vi "Read System Status.vi"(8 "Error in":errorcluster caption="错误输入", 10 "Channel":dbl=1.0 caption="设备通道", 11 "Modbus master in":refnum<class "Modbus Master.lvclass"> caption="Modbus实例输入") -> (0 "Error out":errorcluster caption="错误输出", 1 "Run Status Information":string caption="运行状态信息", 2 "Error Information":string caption="错误信息", 3 "Modbus instance out":refnum<class "Modbus API.lvclass"> caption="Modbus实例输出")   [LabVIEW 2023, in "Longer Pump dLSP501 Series.lvlib"]
uses:
  <instrlib>/Longer Pump dLSP501 Modbus RTU Series/Longer Pump dLSP501 Series.lvlib
  <vilib>/NI/Modbus Library/API/Modbus API.lvclass
  <vilib>/NI/Modbus Library/API/Master/Modbus Master.lvclass
  C:/Program Files/National Instruments/LabVIEW 2023/vi.lib/NI/Modbus Library/API/Modbus API.lvclass
panel:
  out "Register Values":u16[](array[numeric]) caption="寄存器值"
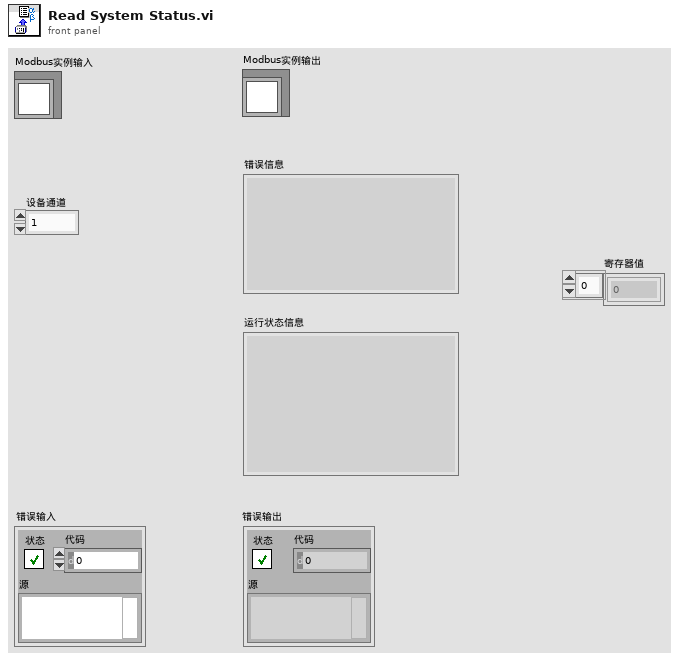
[diagram p1: front panel]
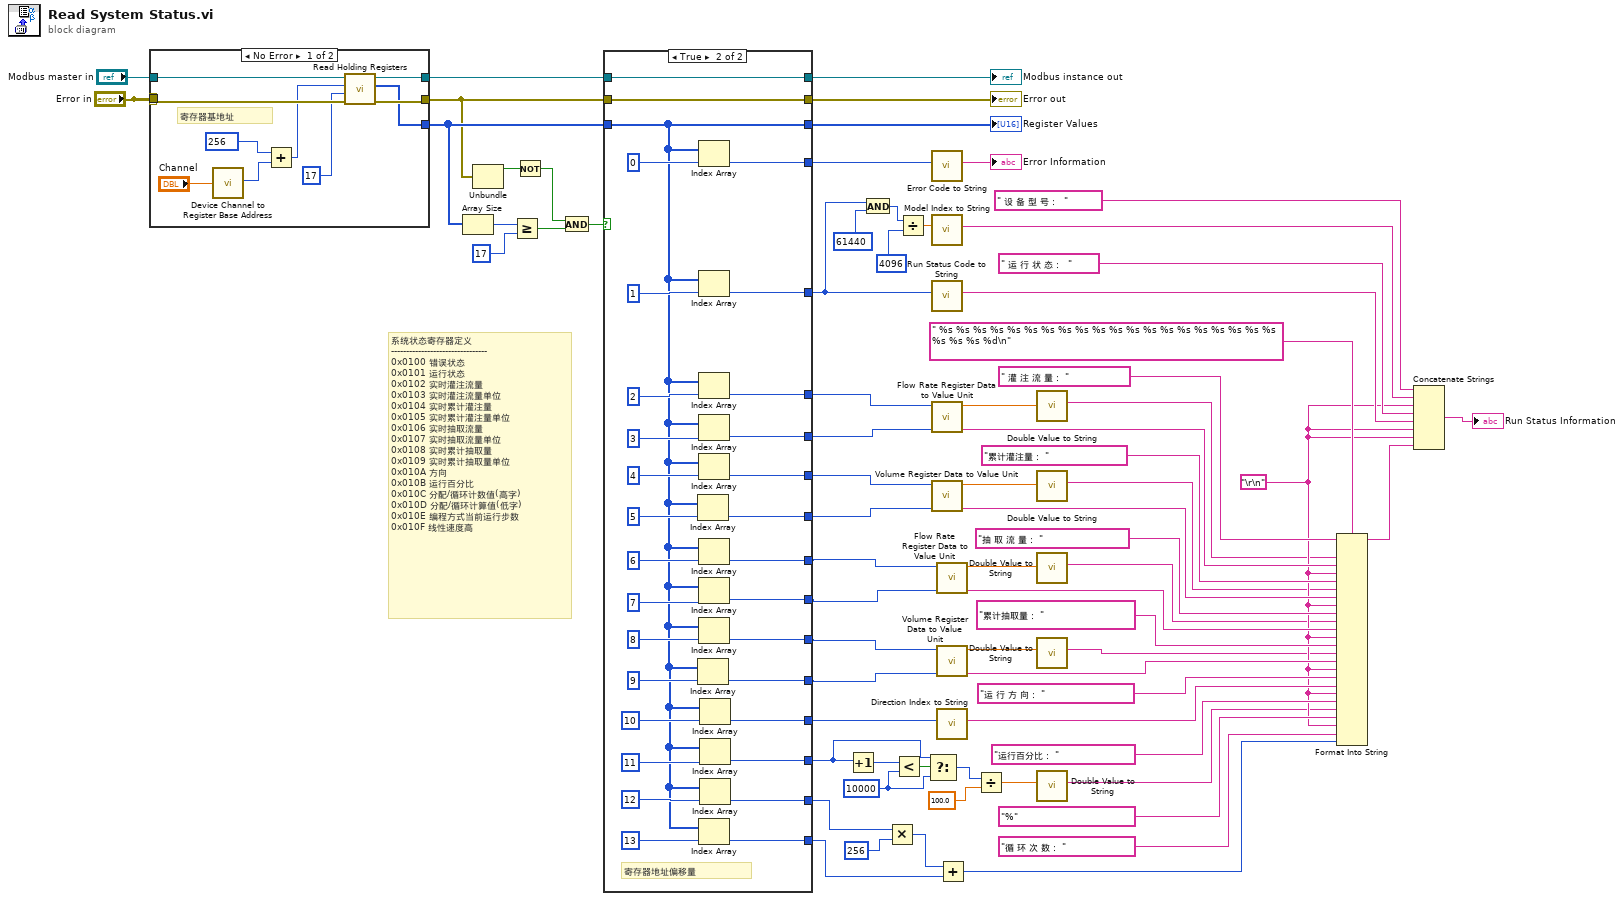
[diagram p0: block diagram]
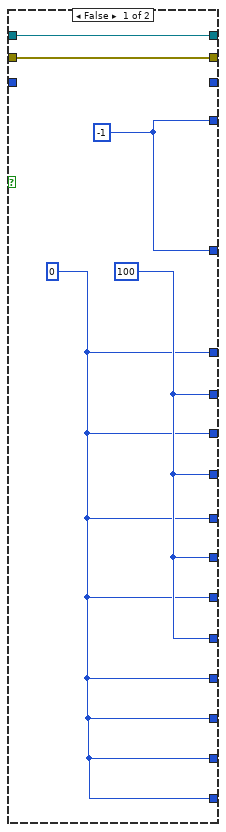
[diagram p2: hidden frame]
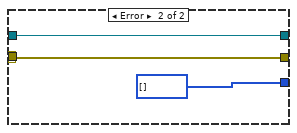
[diagram p3: hidden frame]
diagram:
  w3 = 10000 ("y")
  w31 = "\r\n"
  # "系统状态寄存器定义\n--------------------------------\n0x0100\t错误状态\n0x0101\t运行状态\n0x0102\t实时灌注流量\n0x0103\t实时灌注流量单位\n0x0104\t实时累计灌注量\n0x0105\t实时累计灌注量单位\n0x0106\t实时抽取流量\n0x0107\t实时抽取流量单位\n0x0108\t实时累计抽取量\n0x0109\t实时累计抽取量单位\n0x010A\t方向\n0x010B\t运行百分比\n0x010C\t分配/循环计数值(高字)\n0x010D\t分配/循环计算值(低字)\n0x010E\t编程方式当前运行步数\n0x010F\t线性速度高"
  n1 = case shown="No Error" "Error in" {
    selector: "Error in" -> [_ w85]
    tunnel: "Error in" -> [w82 _]
    tunnel: [w81 w85] -> w18
    tunnel: [w80 w84] -> w71
    tunnel: "Modbus master in" -> [w79 w84]
    tunnel: [w77 u16[] [] ("register values")] -> w22
    frame No Error {
      # "寄存器基地址"
      n2 = call <instrlib>:"Device Channel to Register Base Address.vi"("Channel"="Channel") -> ("Register Base Address"=w75:u16)  [unwired: 10 in]
      n3 = Add(x=u16 256 ("address"), y=w75) -> (x+y=w73:u16)
      n4 = call-dynamic "Read Holding Registers.vi"("error in"=w82, "number of inputs"=u16 17 ("address"), "starting address"=w73, "Modbus master in"=w79) -> ("error out"=w81:errorcluster, "register values"=w77:u16[], "Modbus master out"=w80:refnum<class "Modbus Master.lvclass">)  [unwired: 5 in]
    }
    frame Error {
    }
  }
  n5 = Array Size(array=w22) -> (size(s)=w24:i32)
  n6 = Unbundle(w18) -> ("status"=w21:bool)  [unwired: 2 out]
  n7 = Greater Or Equal?(x=w24, y=17) -> (x >= y?=w25:bool)
  n8 = Not(x=w21) -> (.not. x?=w20:bool)
  n9 = And(x=w20, y=w25) -> (x .and. y?=w19:bool)
  n10 = case shown="True" w19 {
    tunnel: w71 -> [w90 w119]
    tunnel: [w90 w119] -> w70
    tunnel: [w86 w91] -> w16
    tunnel: w22 -> [_ w96]
    tunnel: [w89 w120] -> w34
    tunnel: [w89 w118] -> w27
    tunnel: [w87 w117] -> w67
    tunnel: [w88 w116] -> w66
    tunnel: [_ w96] -> w68
    tunnel: [w87 w112] -> w65
    tunnel: [w88 w111] -> w64
    tunnel: [w87 w104] -> w57
    tunnel: [w88 w103] -> w56
    tunnel: [w87 w102] -> w55
    tunnel: [w88 w101] -> w54
    tunnel: [w87 w95] -> w48
    tunnel: [w87 w94] -> w2
    tunnel: [w87 w93] -> w40
    tunnel: [w87 w92] -> w41
    tunnel: w18 -> [w86 w91]
    frame False {
      w88 = 100
      w87 = 0
      w89 = -1
    }
    frame True {
      # "寄存器地址偏移量"
      n11 = Index Array(array=w96, index=5 ("索引 2")) -> (element=w111:u16)
      n12 = Index Array(array=w96, index=9 ("索引 2")) -> (element=w101:u16)
      n13 = Index Array(array=w96, index=u16 0 ("元素")) -> (element=w120:u16)
      n14 = Index Array(array=w96, index=u16 1 ("元素")) -> (element=w118:u16)
      n15 = Index Array(array=w96, index=2 ("索引")) -> (element=w117:u16)
      n16 = Index Array(array=w96, index=3 ("索引")) -> (element=w116:u16)
      n17 = Index Array(array=w96, index=4 ("索引")) -> (element=w112:u16)
      n18 = Index Array(array=w96, index=6 ("索引")) -> (element=w104:u16)
      n19 = Index Array(array=w96, index=7 ("索引")) -> (element=w103:u16)
      n20 = Index Array(array=w96, index=8 ("索引")) -> (element=w102:u16)
      n21 = Index Array(array=w96, index=13 ("索引 2")) -> (element=w92:u16)
      n22 = Index Array(array=w96, index=10 ("索引")) -> (element=w95:u16)
      n23 = Index Array(array=w96, index=11 ("索引")) -> (element=w94:u16)
      n24 = Index Array(array=w96, index=12 ("索引")) -> (element=w93:u16)
    }
  }
  "Modbus instance out" <- w70
  "Register Values" <- w68
  "Error out" <- w16
  n25 = Increment(x=w2) -> (x+1=w1:i32)
  n26 = And(x=w27, y=u16 61440 ("x与y？")) -> (x .and. y?=w29:i32)
  n27 = Multiply(x=w40, y=256) -> (x*y=w42:i32)
  n28 = Less?(x=w1, y=w3) -> (x < y?=w5:bool)
  n29 = Divide(x=w29, y=u16 4096) -> (x/y=w26:dbl)
  n30 = Select(t=w2, s=w5, f=w3) -> (s? t:f=w4:i32)
  n31 = call <instrlib>:"Error Code to String.vi"("Code"=w34) -> ("Info String"=→"Error Information":string)  [unwired: 10 in]
  n32 = call <instrlib>:"Model Index to String.vi"("Code"=w26) -> ("Info String"=w32:string)  [unwired: 10 in]
  n33 = call <instrlib>:"Run Status Code to String.vi"("Code"=w27) -> ("Info String"=w37:string)  [unwired: 10 in]
  n34 = call <instrlib>:"Flow Rate Register Data to Value Unit.vi"("Value Reg Data"=w67, "Unit Reg Data"=w66) -> ("Flow Rate Value"=w15:dbl, "Flow Rate Unit"=w59:string)  [unwired: 7 in]
  n35 = call <instrlib>:"Volume Register Data to Value Unit.vi"("Value Reg Data"=w65, "Unit Reg Data"=w64) -> ("Volume Value"=w13:dbl, "Volume Unit"=w58:string)  [unwired: 7 in]
  n36 = call <instrlib>:"Flow Rate Register Data to Value Unit.vi"("Value Reg Data"=w57, "Unit Reg Data"=w56) -> ("Flow Rate Value"=w11:dbl, "Flow Rate Unit"=w52:string)  [unwired: 7 in]
  n37 = call <instrlib>:"Volume Register Data to Value Unit.vi"("Value Reg Data"=w55, "Unit Reg Data"=w54) -> ("Volume Value"=w9:dbl, "Volume Unit"=w50:string)  [unwired: 7 in]
  n38 = call <instrlib>:"Direction Index to String.vi"("Value"=w48) -> ("Direction String"=w47:string)  [unwired: 10 in]
  n39 = Add(x=w42, y=w41) -> (x+y=w38:i32)
  n40 = Divide(x=w4, y=100.0) -> (x/y=w7:dbl)
  n41 = call <instrlib>:"Double Value to String.vi"("Value"=w15) -> ("String"=w14:string)  [unwired: 10 in]
  n42 = call <instrlib>:"Double Value to String.vi"("Value"=w13) -> ("String"=w12:string)  [unwired: 10 in]
  n43 = call <instrlib>:"Double Value to String.vi"("Value"=w11) -> ("String"=w10:string)  [unwired: 10 in]
  n44 = call <instrlib>:"Double Value to String.vi"("Value"=w9) -> ("String"=w8:string)  [unwired: 10 in]
  n45 = call <instrlib>:"Double Value to String.vi"("Value"=w7) -> ("String"=w6:string)  [unwired: 10 in]
  n46 = Format Into String(format string=" %s %s %s %s %s %s %s %s %s %s %s %s %s %s %s %s %s %s %s %s %s %s %s %d\n", initial string=" 灌 注 流 量： ", w14, w59, w31, "累计灌注量： ", w12, w58, w31, "抽 取 流 量： ", w10, w52, w31, "累计抽取量： ", w8, w50, w31, "运 行 方 向： ", w47, w31, "运行百分比： ", w6, "%", w31, "循 环 次 数： ", w38) -> (resulting string=w35:string)  [unwired: 1 in, 1 out]
  n47 = Concatenate Strings(" 设 备 型 号：  ", w32, w31, " 运 行 状 态：  ", w37, w31, w31, w35) -> (→"Run Status Information":string)
